vi "Cleanup.vi"(8 "error in (no error)":errorcluster, 11 "Flex  Dialog (Actor) in":refnum<class "Flex Dialog (Actor).lvclass">) -> (0 "error out":errorcluster, 3 "Flex  Dialog (Actor) out":refnum<class "Flex Dialog (Actor).lvclass">)   [LabVIEW 2014, in "Flex UI Dialog (Actor).lvlib" / "Flex Dialog (Actor).lvclass"]
uses:
  Flex Dialog (Actor).lvclass
  Flex UI (Actor)/Flex UI (Actor).lvclass
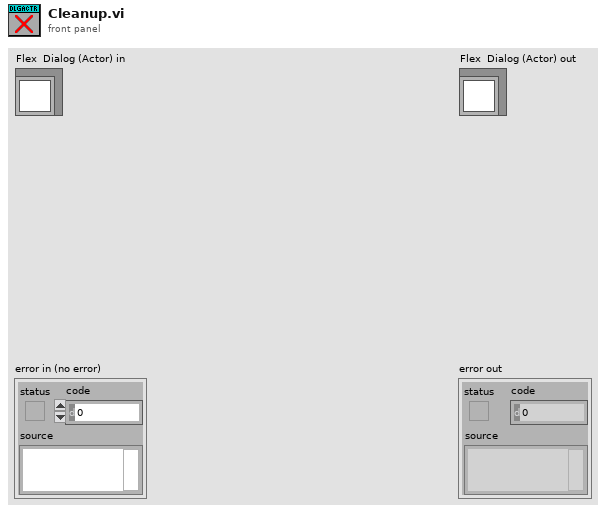
[diagram p1: front panel]
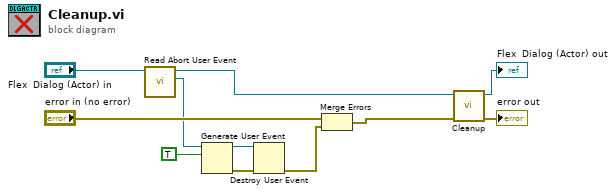
[diagram p0: block diagram]
diagram:
  n1 = call-dynamic "Read Abort User Event.vi"("Flex  Dialog (Actor) in"="Flex  Dialog (Actor) in") -> ("Abort User Event"=w5:refnum<user-event>, "Flex  Dialog (Actor) out"=w3:refnum<class "Flex Dialog (Actor).lvclass">)  [unwired: 9 in]
  n2 = Generate User Event(user event=w5, event data cluster=TRUE ("event data")) -> (user event out=w8:refnum<user-event>, error out=w7:errorcluster)  [unwired: 2 in]
  n3 = Destroy User Event(user event=w8, error in=w7) -> (error out=w1:errorcluster)
  n4 = Merge Errors("error in (no error)", w1) -> (w2:errorcluster)
  n5 = call-parent "Cleanup.vi"("error in (no error)"=w2, "Flex UI (Actor) in"=w3) -> ("error out"=→"error out":errorcluster, "Flex UI (Actor) out"=→"Flex  Dialog (Actor) out":refnum<class "Flex Dialog (Actor).lvclass">)  [unwired: 8 in]
